vi "Test Import Control Names.vi"() -> ()   [LabVIEW 2013, in "FPGA Module tests.lvlib"]
uses:
  FPGA Module tests.lvlib
  <vilib>/rvi/interface/common/nirviReadCallControlInfo.ctl
panel:
  in  "bitfile path":path
  out "controls":T1
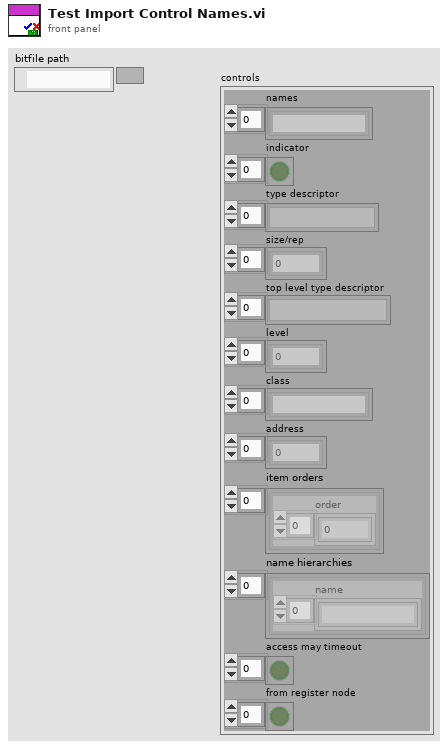
[diagram p1: front panel]
types:
  T1 = typedef "nirviReadCallControlInfo.ctl" = cluster{"names":string[], "indicator":bool[], "type descriptor":variant[], "size/rep":u32[], "top level type descriptor":variant[], "level":i32[], "class":string[], "address":i32[], "item orders":cluster{"order":u32[]}[], "name hierarchies":cluster{"name":string[]}[], "access may timeout":bool[], "from register node":bool[]}
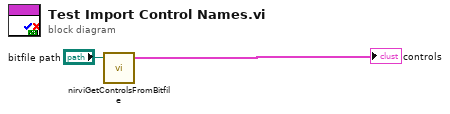
[diagram p0: block diagram]
diagram:
  n1 = call <vilib>:"nirviGetControlsFromBitfile.vi"("bitfile path"="bitfile path") -> ("controls"=→"controls":T1)  [unwired: 3 in, 1 out]
